vi "p5.3 (hw4).vi"() -> ()   [LabVIEW 2017]
panel:
  out "Average of last 4":dbl
  in  "Press to Stop":bool
  out "Random Number":dbl
  # "P5.3"
  # "Patrik Sokolowski"
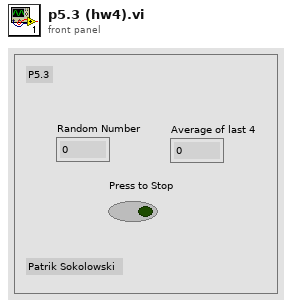
[diagram p1: front panel]
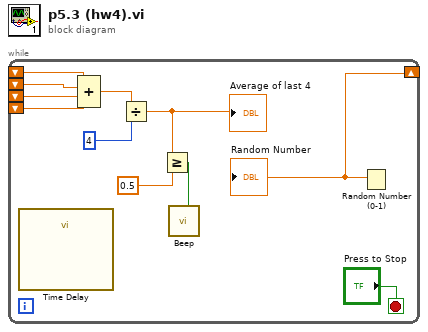
[diagram p0: block diagram]
diagram:
  n1 = while {
    shift-right: [w8] -> _
    shift-left: _ -> [w7]
    shift-left: _ -> [w6]
    shift-left: _ -> [w5]
    shift-left: _ -> [w4]
    stop <- "Press to Stop" stop-if-true
    n2 = call "Time Delay"() -> ()  [unwired: 11 in, 1 out]
    n3 = Compound Arithmetic op=ADD(w7, w6, w5, w4) -> (w9:dbl)
    n4 = Divide(x=w9, y=4) -> (x/y=w3:dbl)
    "Average of last 4" <- w3
    n5 = Greater Or Equal?(x=w3, y=0.5) -> (x >= y?=w1:bool)
    n6 = call <vilib>:"Beep.vi"("use system alert? (T)"=w1) -> ()  [unwired: 11 in]
    n7 = Random Number (0-1)() -> (number: 0 to 1=w8:dbl)
    "Random Number" <- w8
  }
